vi "WLAN_RSMA_FrameBuild - 3 SC.vi"(5 "Beta/Alpha":dbl min=0.0 max=1.0 step=0.05 format="%#_13g", 7 "Alpha":dbl min=0.0 max=1.0 step=0.05 format="%#_13g", 8 "error in (no error)":errorcluster, 9 "data in 2":i8[](array[numeric]) caption="input bit stream", 10 "Modulation parameter":T2, 11 "data in":i8[](array[numeric]) caption="input bit stream") -> (0 "error out":errorcluster, 3 "output array":cdb[](array[numeric]))   [LabVIEW 2022 SP3]
panel:
  in  "Modulation type 2":T1(ring)=enum."BPSK Vertical"
  in  "Modulation type":enum16{"QPSK(4QAM)", "64QAM", "16QAM", "BPSK"}(ring)=enum."BPSK"
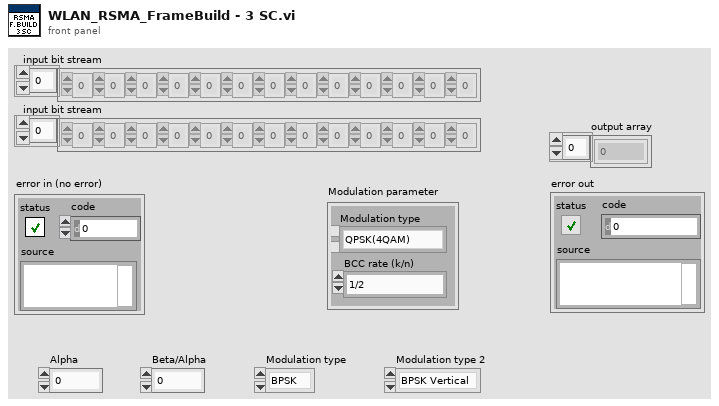
[diagram p1: front panel]
types:
  T1 = enum16{"QPSK(4QAM)", "64QAM", "16QAM", "BPSK", "BPSK Vertical"}
  T2 = cluster{"Modulation type":enum16{"QPSK(4QAM)", "64QAM", "16QAM", "BPSK"}, "BCC rate (k/n)":enum16{"1/2", "2/3", "3/4"}}
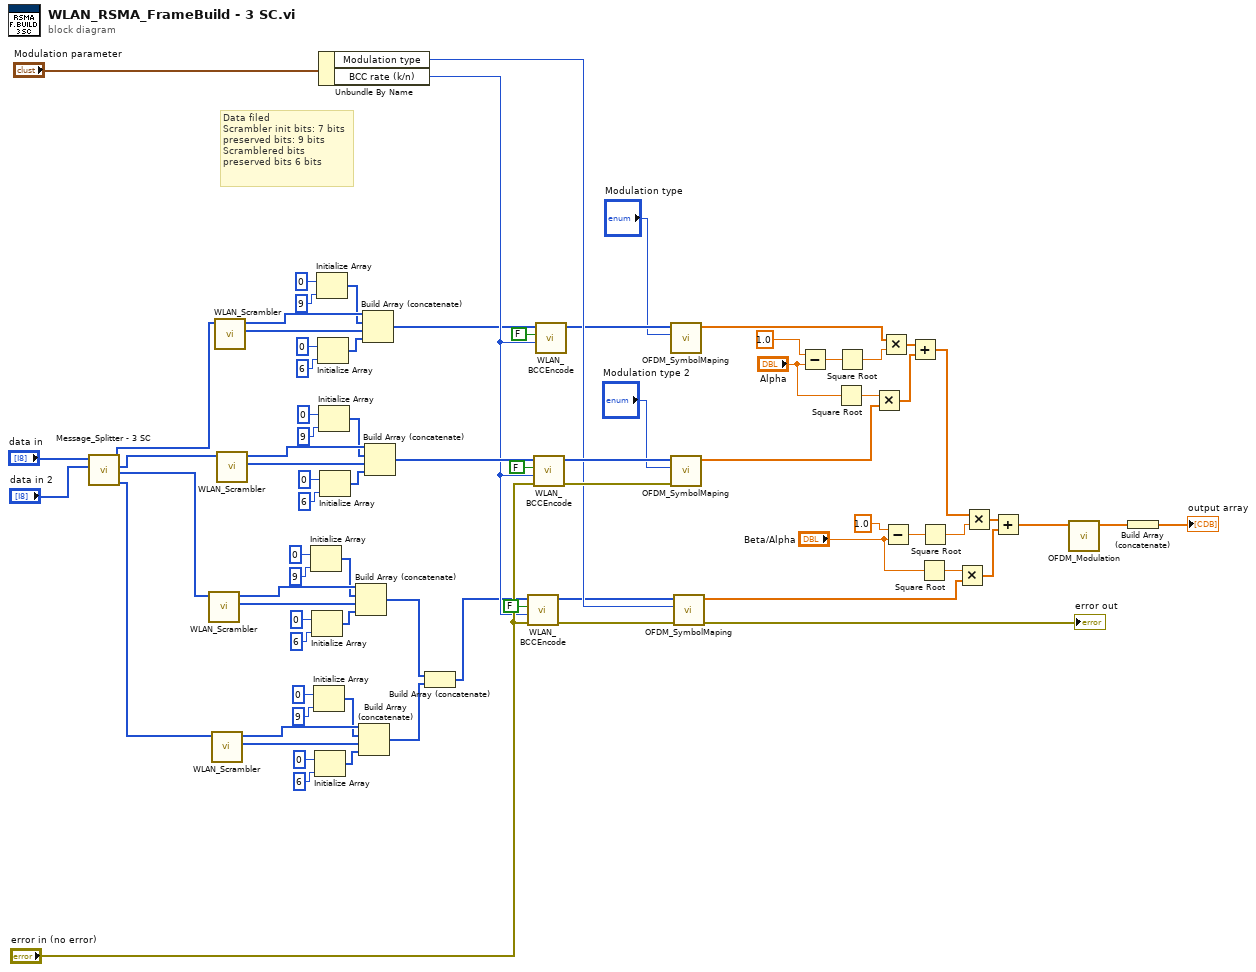
[diagram p0: block diagram]
diagram:
  # "Data filed\nScrambler init bits: 7 bits\npreserved bits: 9 bits\nScramblered bits\npreserved bits 6 bits"
  n1 = call "Message_Splitter - 3 SC.vi"("W2"="data in 2", "W1"="data in") -> ("Wp2"=w1:u8[], "Wp1"=w2:u8[], "Wc2"=w28:u8[], "Wc1"=w27:u8[])  [unwired: 6 in]
  n2 = call "WLAN_Scrambler.vi"("input bit stream"=w2) -> ("scrambled bits"=w59:i8[], "scrambler initial bit"=w63:i8[])  [unwired: 9 in]
  n3 = call "WLAN_Scrambler.vi"("input bit stream"=w1) -> ("scrambled bits"=w9:i8[], "scrambler initial bit"=w13:i8[])  [unwired: 9 in]
  n4 = call "WLAN_Scrambler.vi"("input bit stream"=w27) -> ("scrambled bits"=w30:i8[], "scrambler initial bit"=w37:i8[])  [unwired: 9 in]
  n5 = call "WLAN_Scrambler.vi"("input bit stream"=w28) -> ("scrambled bits"=w55:i8[], "scrambler initial bit"=w70:i8[])  [unwired: 9 in]
  n6 = Initialize Array(i8 0 ("element"), 9 ("dimension size")) -> (w62:i8[])
  n7 = Initialize Array(i8 0 ("element"), 6 ("dimension size")) -> (w56:i8[])
  n8 = Initialize Array(i8 0 ("element"), 9 ("dimension size")) -> (w12:i8[])
  n9 = Initialize Array(i8 0 ("element"), 6 ("dimension size")) -> (w6:i8[])
  n10 = Initialize Array(i8 0 ("element"), 9 ("dimension size")) -> (w36:i8[])
  n11 = Initialize Array(i8 0 ("element"), 6 ("dimension size")) -> (w31:i8[])
  n12 = Unbundle By Name("Modulation parameter") -> ("Modulation type"=w74:enum16{"QPSK(4QAM)", "64QAM", "16QAM", "BPSK"}, "BCC rate (k/n)"=w25:enum16{"1/2", "2/3", "3/4"})
  n13 = Initialize Array(i8 0 ("element"), 9 ("dimension size")) -> (w69:i8[])
  n14 = Initialize Array(i8 0 ("element"), 6 ("dimension size")) -> (w64:i8[])
  n15 = Build Array (concatenate)(w63, w62, w59, w56) -> (w5:i8[])
  n16 = Build Array (concatenate)(w13, w12, w9, w6) -> (w4:i8[])
  n17 = Build Array (concatenate)(w37, w36, w30, w31) -> (w24:i8[])
  n18 = Build Array (concatenate)(w70, w69, w55, w64) -> (w79:i8[])
  n19 = Build Array (concatenate)(w5, w4) -> (w3:i8[])
  n20 = call "WLAN_BCCEncode.vi"("error in (no error)"="error in (no error)", "BCC rate (k/n)"=w25, "need add zeros?"=FALSE, "input bit stream"=w3) -> ("error out"=w71:errorcluster, "output bit stream 3"=w72:i8[])  [unwired: 6 in]
  n21 = call "WLAN_BCCEncode.vi"("error in (no error)"="error in (no error)", "BCC rate (k/n)"=w25, "need add zeros?"=FALSE, "input bit stream"=w79) -> ("error out"=w77:errorcluster, "output bit stream 3"=w76:i8[])  [unwired: 6 in]
  n22 = call "WLAN_BCCEncode.vi"("BCC rate (k/n)"=w25, "need add zeros?"=FALSE, "input bit stream"=w24) -> ("output bit stream 3"=w23:i8[])  [unwired: 7 in, 1 out]
  n23 = call "OFDM_SymbolMaping.vi"("Modulation type"="Modulation type", "input bit stream"=w23) -> ("symbols"=w18:cdb[])  [unwired: 8 in, 1 out]
  n24 = call "OFDM_SymbolMaping.vi"("error in (no error)"=w77, "Modulation type"="Modulation type 2", "input bit stream"=w76) -> ("symbols"=w19:cdb[])  [unwired: 7 in, 1 out]
  n25 = call "OFDM_SymbolMaping.vi"("error in (no error)"=w71, "Modulation type"=w74, "input bit stream"=w72) -> ("error out"=→"error out":errorcluster, "symbols"=w20:cdb[])  [unwired: 7 in]
  n26 = Subtract(x=1.0, y="Alpha") -> (x-y=w47:dbl)
  n27 = Square Root(x="Alpha") -> (sqrt(x)=w51:dbl)
  n28 = Square Root(x=w47) -> (sqrt(x)=w49:dbl)
  n29 = Multiply(x=w51, y=w19) -> (x*y=w52:cdb[])
  n30 = Multiply(x=w18, y=w49) -> (x*y=w50:cdb[])
  n31 = Subtract(x=1.0, y="Beta/Alpha") -> (x-y=w38:dbl)
  n32 = Add(x=w50, y=w52) -> (x+y=w17:cdb[])
  n33 = Square Root(x="Beta/Alpha") -> (sqrt(x)=w41:dbl)
  n34 = Square Root(x=w38) -> (sqrt(x)=w39:dbl)
  n35 = Multiply(x=w41, y=w20) -> (x*y=w42:cdb[])
  n36 = Multiply(x=w17, y=w39) -> (x*y=w40:cdb[])
  n37 = Add(x=w40, y=w42) -> (x+y=w16:cdb[])
  n38 = call "OFDM_Modulation.vi"("Input sequence"=w16) -> ("Output sequence"=w45:cdb[])  [unwired: 10 in]
  n39 = Build Array (concatenate)(w45) -> (→"output array":cdb[])
